vi "Get Queue Status.vi"(8 "error in (no error)":errorcluster, 9 "return elements? (T)":bool=TRUE, 11 "Message Queue":T1) -> (0 "error out":errorcluster, 2 "Queue Status":T2, 3 "queue out":T1)   [LabVIEW 2019, in "Task Manager.lvlib"]
uses:
  Task Manager.lvlib
  Shared/TypeDefs/Message Queue Ref.ctl
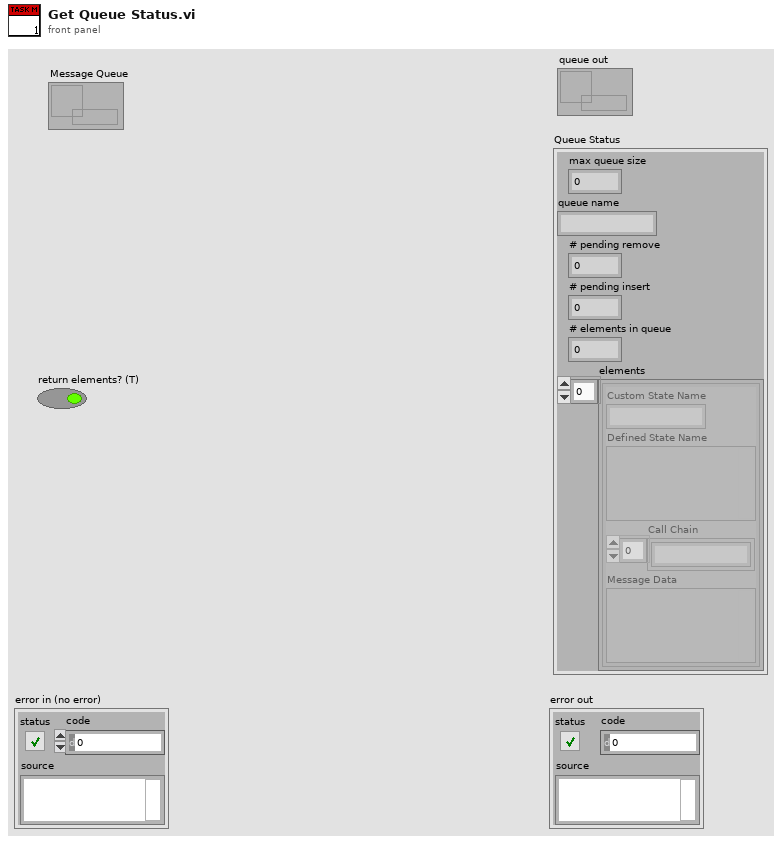
[diagram p1: front panel]
types:
  T1 = typedef "Message Queue Ref.ctl" = refnum<queue>
  T2 = cluster{"max queue size":i32, "queue name":string, "# pending remove":i32, "# pending insert":i32, "# elements in queue":i32, "elements":cluster{"Custom State Name":string, "Defined State Name":variant, "Call Chain":string[], "Message Data":variant}[]}
  T3 = cluster{"Custom State Name":string, "Defined State Name":variant, "Call Chain":string[], "Message Data":variant}[]
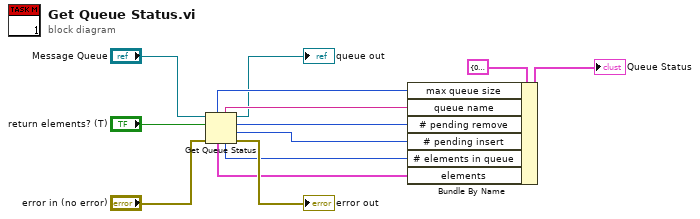
[diagram p0: block diagram]
diagram:
  n1 = Get Queue Status(queue="Message Queue", return elements? (F)="return elements? (T)", error in (no error)="error in (no error)") -> (queue out=→"queue out":T1, queue name=w7:string, max queue size=w8:i32, # pending remove=w6:i32, # pending insert=w1:i32, error out=→"error out":errorcluster, # elements in queue=w5:i32, elements=w4:T3)
  n2 = Bundle By Name(cluster=T2 {"max queue size"=0, "queue name"="", "# pending remove"=0, "# pending insert"=0, "# elements in queue"=0, "elements"=[]} ("Queue Status"), "max queue size"=w8, "queue name"=w7, "# pending remove"=w6, "# pending insert"=w1, "# elements in queue"=w5, "elements"=w4) -> (→"Queue Status":T2)
